vi "Read Debug info.vi"(11 "CDebugInfo in":refnum<class "CDebugInfo.lvclass">) -> (1 "Debug info":string, 3 "CDebugInfo out":refnum<class "CDebugInfo.lvclass">)   [LabVIEW 2020, in "DependencyInspection.lvlib" / "CDebugInfo.lvclass"]
uses:
  CDebugInfo.lvclass
  CDebugInfo.lvclass/CDebugInfo.ctl
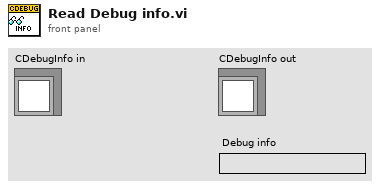
[diagram p1: front panel]
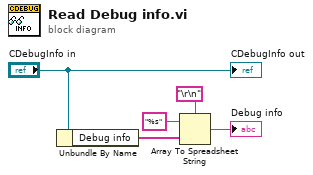
[diagram p0: block diagram]
diagram:
  n1 = Unbundle By Name("CDebugInfo in") -> ("Debug info"=w2:string[])
  n2 = Array To Spreadsheet String(delimiter (Tab)="\r\n", array=w2, 3:"%s" ("format string")) -> (spreadsheet string=→"Debug info":string)
  "CDebugInfo out" <- "CDebugInfo in"
